vi "Query SigGen Amplitude.vi"(7 "Frequency":dbl, 8 "error in (no error)":errorcluster, 9 "Cal?":bool, 10 "Cal Route":string[](array[string]), 11 "VISA In":refnum<visa-resource-name>) -> (0 "error out":errorcluster, 2 "Amplitude (dBm)":dbl format="%_4f", 3 "VISA Out":refnum<visa-resource-name>)   [LabVIEW 2015]
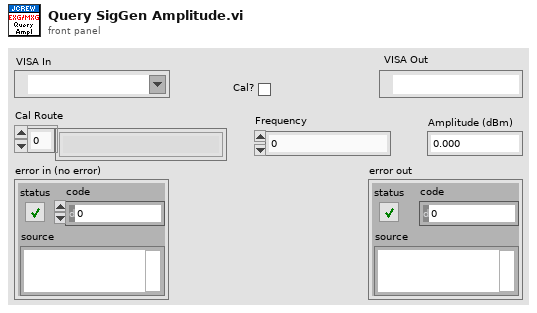
[diagram p1: front panel]
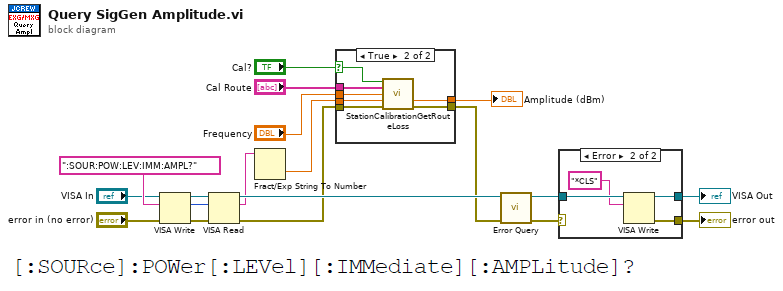
[diagram p0: block diagram]
diagram:
  n1 = VISA Write(VISA resource name="VISA In", write buffer=":SOUR:POW:LEV:IMM:AMPL?", error in (no error)="error in (no error)") -> (VISA resource name out=w15:refnum<visa-resource-name>, return count=w19:u32, error out=w14:errorcluster)
  n2 = VISA Read(VISA resource name=w15, byte count=w19, error in (no error)=w14) -> (VISA resource name out=w12:refnum<visa-resource-name>, read buffer=w8:string, error out=w4:errorcluster)  [unwired: 1 out]
  n3 = Fract/Exp String To Number(string=w8) -> (number=w6:dbl)  [unwired: 3 in, 1 out]
  n4 = case shown="True" "Cal?" {
    selector: "Cal?" -> [_ w22]
    tunnel: [w20 w28] -> w7
    tunnel: [w21 w23] -> w1
    tunnel: w4 -> [w21 w27]
    tunnel: w6 -> [w20 w26]
    tunnel: "Cal Route" -> [_ w25]
    tunnel: "Frequency" -> [_ w24]
    frame False {
    }
    frame True {
      n5 = call "StationCalibrationGetRouteLoss.vi"("Calibration Enabled"=w22, "Route Names"=w25, "Frequency"=w24, "Power Level"=w26, "error in (no error)"=w27) -> ("Adjusted Power Level"=w28:dbl, "error out"=w23:errorcluster)  [unwired: 7 in, 2 out]
    }
  }
  "Amplitude (dBm)" <- w7
  n6 = call <instrlib>:"Error Query.vi"("error in (no error)"=w1, "VISA resource name"=w12) -> ("error out"=w9:errorcluster, "VISA resource name out"=w11:refnum<visa-resource-name>)  [unwired: 6 in, 2 out]
  n7 = case shown="Error" w9 {
    selector: w9 -> [w30 _]
    tunnel: [w29 w34] -> w13
    tunnel: w11 -> [w29 w33]
    tunnel: [w30 w32] -> w10
    frame No Error {
    }
    frame Error {
      n8 = VISA Write(VISA resource name=w33, write buffer="*CLS") -> (VISA resource name out=w34:refnum<visa-resource-name>, error out=w32:errorcluster)  [unwired: 1 in, 1 out]
    }
  }
  "VISA Out" <- w13
  "error out" <- w10
